vi "Call_LockinIV.vi"(11 "Channels: AO in":T1) -> ()   [LabVIEW 2013]
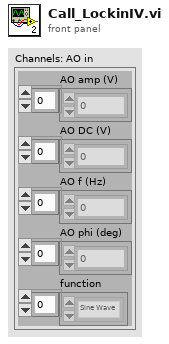
[diagram p1: front panel]
types:
  T1 = cluster{"AO amp (V)":dbl[], "AO DC (V)":dbl[], "AO f (Hz)":dbl[], "AO phi (deg)":dbl[], "function":enum16{"Sine Wave", "Triangle Wave", "Square Wave", "Sawtooth Wave"}[]}
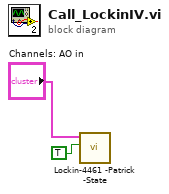
[diagram p0: block diagram]
diagram:
  n1 = call <userlib>:"Lockin-4461 -Patrick -State.vi"("IV Curve Mode"=TRUE, "Channels: AO"="Channels: AO in") -> ()  [unwired: 10 in]
